vi "VI_B.vi"() -> ()   [LabVIEW 2013]
uses:
  stop_B.vi
  stop_A.vi
panel:
  out "numeri che hanno\nbloccato VI_A":string[](array[string])
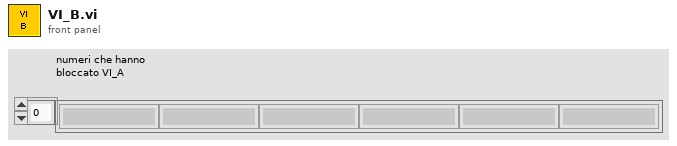
[diagram p1: front panel]
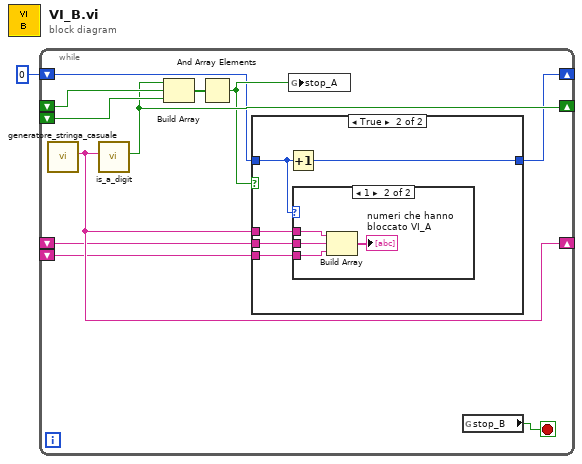
[diagram p0: block diagram]
diagram:
  n1 = while {
    shift-right: [w8] -> _
    shift-left: _ -> [w12]
    shift-left: _ -> [w11]
    shift-right: [w6] -> _
    shift-left: _ -> [w5]
    shift-left: _ -> [w4]
    shift-right: [w2] -> _
    shift-left: 0 -> [w3]
    stop <- w9 stop-if-true
    n2 = call "generatore_stringa_casuale.vi"() -> ("stringa"=w6:string)  [unwired: 11 in]
    n3 = call "is_a_digit.vi"("String"=w6) -> ("is a digit"=w8:bool)  [unwired: 10 in]
    n4 = Build Array(w8, w12, w11) -> (w10:bool[])
    n5 = And Array Elements(Boolean array=w10) -> (logical AND=w7:bool)
    n6 = case shown="True" w7 {
      tunnel: w6 -> [_ w18]
      tunnel: w5 -> [_ w17]
      tunnel: w4 -> [_ w16]
      tunnel: w3 -> [w13 w15]
      tunnel: [w13 w14] -> w2
      frame False {
      }
      frame True {
        n7 = Increment(x=w15) -> (x+1=w14:i32)
        n8 = case shown="1" w15 {
          tunnel: w18 -> [_ w22]
          tunnel: w17 -> [_ w21]
          tunnel: w16 -> [_ w20]
          frame 0, Default {
          }
          frame 1 {
            n9 = Build Array(w22, w21, w20) -> (→"numeri che hanno\nbloccato VI_A":string[])
          }
        }
      }
    }
    n10 = global write "stop_A.vi" "stop_A"(w7) -> ()
    n11 = global read "stop_B.vi" "stop_B"() -> (w9:bool)
  }
